vi "VI-File-Explorer_1.vi"() -> ()   [LabVIEW 2021, in "vi_lib.lvlib"]
uses:
  vi_lib.lvlib
  clLabview/clLabview.lvclass
  clFile/clFile.lvclass
panel:
  out "concatenated string":string
  in  "new VI-Lib Password":string
  in  "Update LV-Lib Password":bool
  out "File is protected?":bool=TRUE
  out "LV-Lib password (Hex)":string
  out "Icon":picture
  out "busy (*)":bool
  out "Salt (Hex)":string
  out "MD5-Hash 2 (Hex)":string
  out "MD5-Hash 1 (Hex)":string
  out "saving done":bool
  in  "save":bool
  in  "Open":bool
  in  "stop":bool
  out "flags":i32 step=1
  out "stage":u8(ring) items=["development", "alpha", "beta", "release"]
  out "build":u8 step=1
  out "bugfix":u8 step=1
  out "minor":u8 max=99 step=1
  out "major":u8=3 min=1 max=99 step=1
  out "version info":string
  out "version text":string
  in  "save to":path=path "D:/labview/file_in_(free).vi"
  in  "new File Password":string
  in  "open from":path=path "D:/labview/file.vi"
  out "MD5 password (Hex)":string
  # "MD5 password (Hex)\nMD5-Hash 1 (Hex)\nMD5-Hash 2 (Hex) for LV-Version >= 8\nLV-Lib password (Hex)"
  # "File password [BDPW]"
  # "for LV-Version >= 8"
  # "for LV-Version >= 12"
  # "File propertys [LVSR]"
  # "(*) This is a \"brute force\" version to calc the password Salt, \n      so it might take up to 30sec."
  # "File version [vers]"
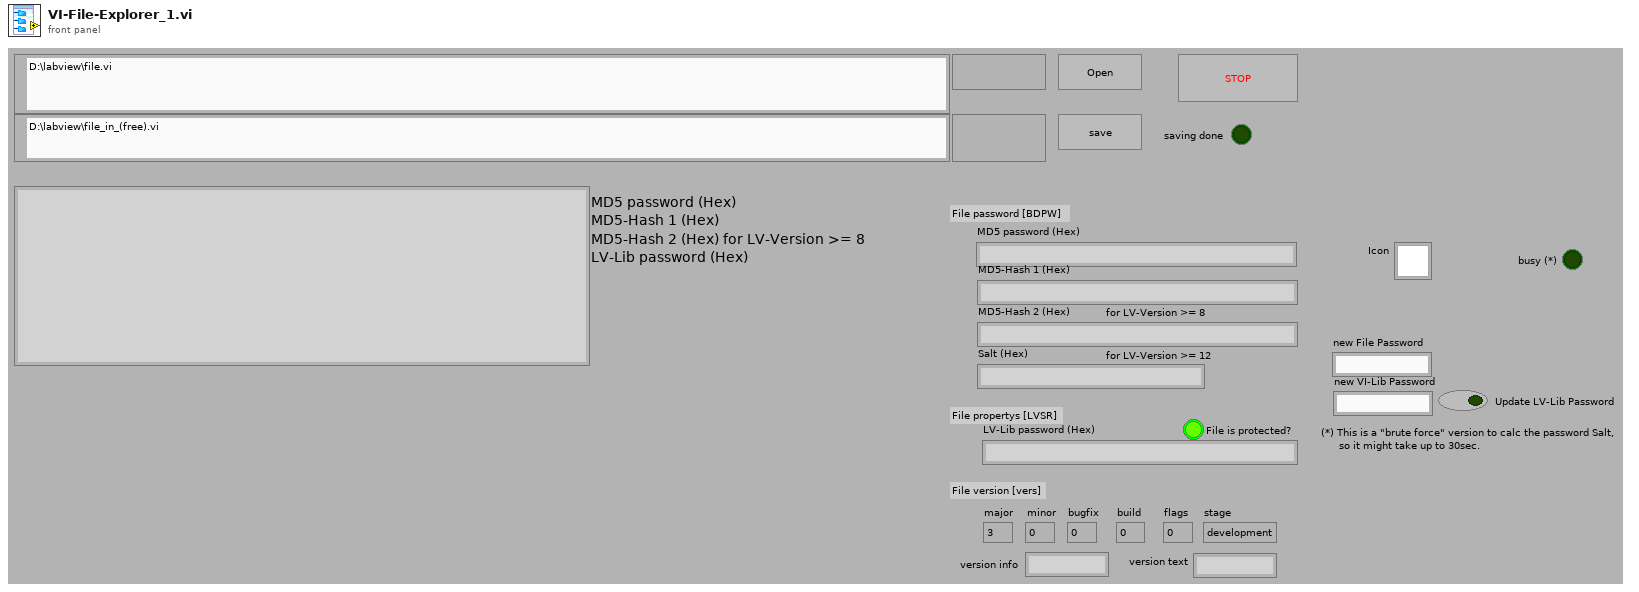
[diagram p1: front panel]
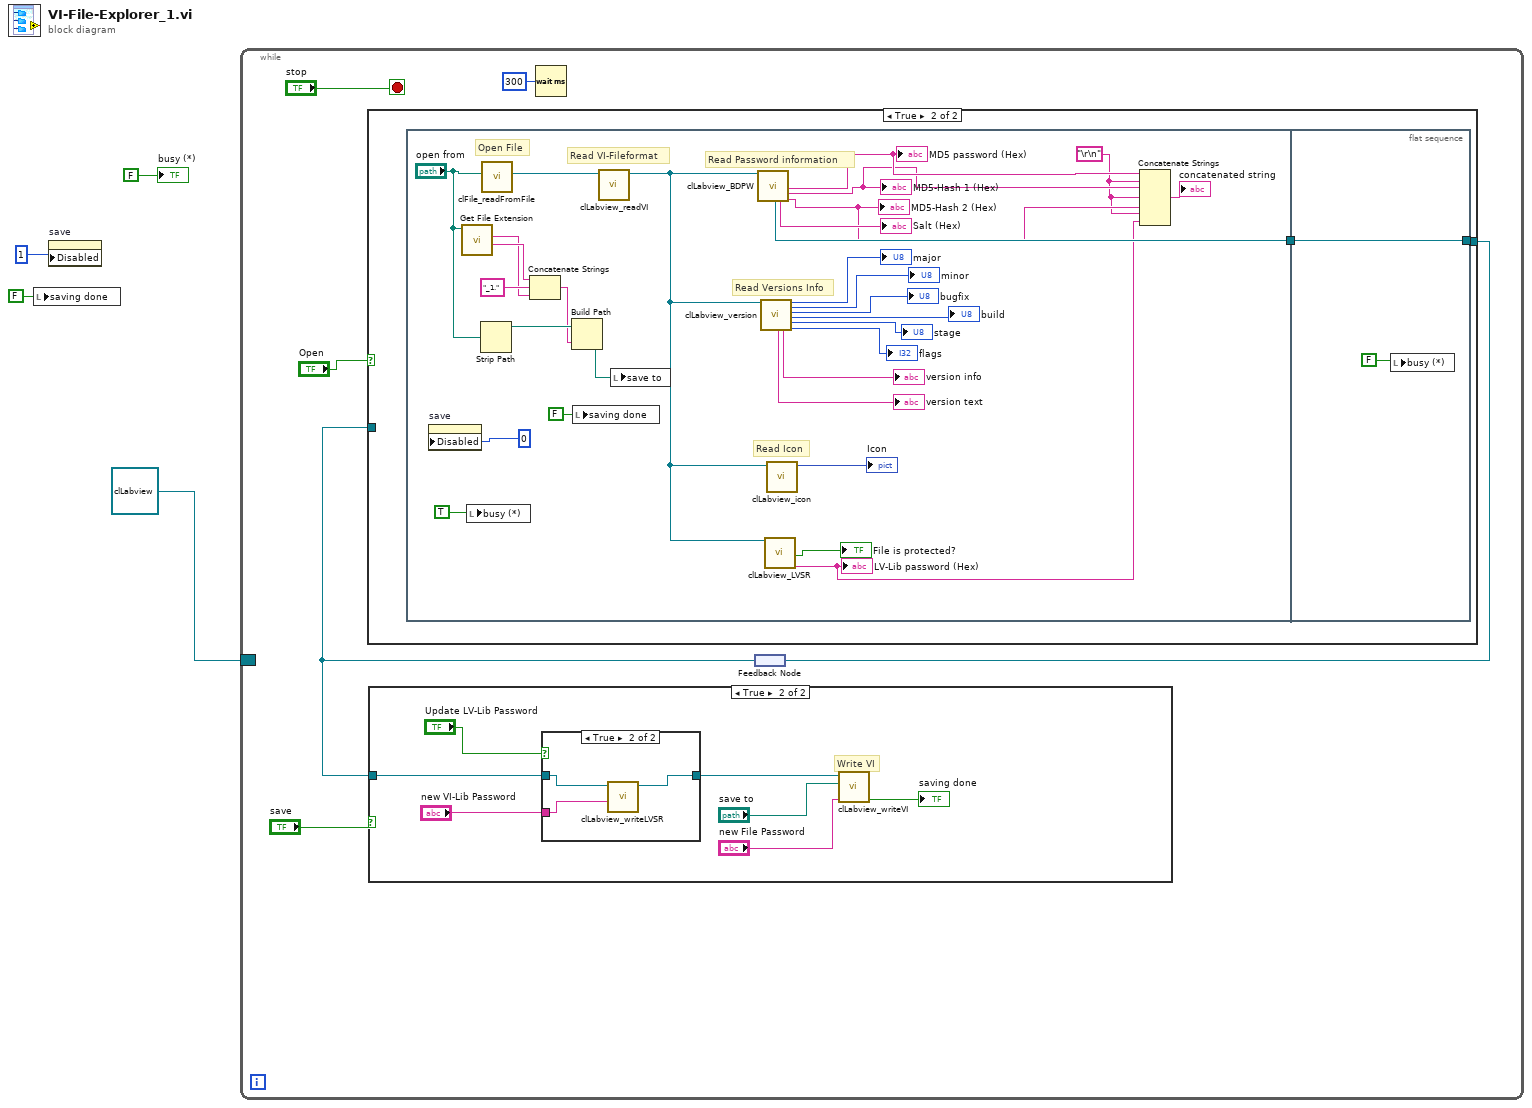
[diagram p0: block diagram]
diagram:
  n1 = local write "saving done"(FALSE ("saving done")) -> ()
  n2 = property on="save" class="Bool"("Disabled"=u8 1) -> ()  [unwired: 2 in, 2 out]
  n3 = while {
    border: refnum<class "clLabview.lvclass"> refnum ("vi_lib.lvlib:clLabview.lvclass 2") -> [_]
    stop <- "stop" stop-if-true
    n4 = Wait (ms)(milliseconds to wait=u32 300) -> ()  [unwired: 1 out]
    n5 = feedback #1() -> (w6:refnum<class "clLabview.lvclass">)
    n6 = case shown="True" "Open" {
      tunnel: [w22 w24] -> w8
      tunnel: w6 -> [w22 _]
      frame False {
      }
      frame True {
        n7 = flat-sequence {
          tunnel: [w43] -> w23
          tunnel: [w56] -> w24
          tunnel: w23 -> [w56]
          frame #0 {
            w27 = "\r\n"
            # "Read Icon"
            # "Read Versions Info"
            # "Read Password information"
            # "Read VI-Fileformat"
            # "Open File"
            n8 = property on="save" class="Bool"("Disabled"=u8 0) -> ()  [unwired: 2 in, 2 out]
            n9 = call <vilib>:"Get File Extension.vi"("file"="open from") -> ("filename without extension"=w35:string, "lowercase file extension"=w33:string)  [unwired: 6 in, 3 out]
            n10 = local write "busy (*)"(TRUE ("busy")) -> ()
            n11 = Strip Path(path="open from") -> (stripped path=w37:path)  [unwired: 1 out]
            n12 = call "clFile_readFromFile.vi"("file (use dialog)"="open from") -> ("clFileReader.lvclass"=w54:refnum<class "clFileReader.lvclass">)  [unwired: 1 in, 9 out]
            n13 = Concatenate Strings(w35, "_1." ("string"), w33) -> (w32:string)
            n14 = Build Path(base path=w37, name or relative path=w32) -> (appended path=w36:path)
            n15 = local write "saving done"(FALSE ("saving done")) -> ()
            n16 = call "clLabview_readVI.vi"("vi_lib.lvlib:clFileReader.lvclass"=w54) -> ("vi_lib.lvlib:clLabview.lvclass 2"=w40:refnum<class "clLabview.lvclass">)  [unwired: 10 out]
            n17 = local write "save to"(w36) -> ()
            n18 = call "clLabview_BDPW.vi"("vi_lib.lvlib:clLabview.lvclass"=w40) -> ("vi_lib.lvlib:clLabview.lvclass [Out]"=w43:refnum<class "clLabview.lvclass">, "Salt (Hex)"=→"Salt (Hex)":string, "MD5 password (Hex)"=w31:string, "MD5-Hash 1  (Hex)"=w30:string, "MD5-Hash 2  (Hex)"=w29:string)  [unwired: 14 out]
            "MD5 password (Hex)" <- w31
            "MD5-Hash 2 (Hex)" <- w29
            "MD5-Hash 1 (Hex)" <- w30
            n19 = call "clLabview_version.vi"("vi_lib.lvlib:clLabview.lvclass"=w40) -> ("version_text"=→"version text":string, "version_info"=→"version info":string, "major"=→"major":u8, "minor"=→"minor":u8, "bugfix"=→"bugfix":u8, "build"=→"build":u8, "stage"=→"stage":u8, "flags"=→"flags":i32)  [unwired: 11 out]
            n20 = call "clLabview_LVSR.vi"("vi_lib.lvlib:clLabview.lvclass"=w40) -> ("File is protected?"=→"File is protected?":bool, "MD5 lib Password (Hex)"=w26:string)  [unwired: 17 out]
            "LV-Lib password (Hex)" <- w26
            n21 = call "clLabview_icon.vi"("vi_lib.lvlib:clLabview.lvclass"=w40) -> ("Icon"=→"Icon":picture)  [unwired: 10 out]
            n22 = Concatenate Strings(w31, w27, w30, w27, w29, w27, w26) -> (→"concatenated string":string)
          }
          frame #1 {
            n23 = local write "busy (*)"(FALSE ("busy")) -> ()
          }
        }
      }
    }
    n24 = case shown="True" "save" {
      tunnel: w6 -> [_ w13]
      frame False {
      }
      frame True {
        # "Write VI"
        n25 = case shown="True" "Update LV-Lib Password" {
          tunnel: w13 -> [w18 w21]
          tunnel: [w18 w20] -> w14
          tunnel: "new VI-Lib Password" -> [_ w19]
          frame False {
          }
          frame True {
            n26 = call "clLabview_writeLVSR.vi"("vi_lib.lvlib:clLabview.lvclass"=w21, "new lib Password"=w19) -> ("vi_lib.lvlib:clLabview.lvclass [Out]"=w20:refnum<class "clLabview.lvclass">)  [unwired: 8 out]
          }
        }
        n27 = call "clLabview_writeVI.vi"("vi_lib.lvlib:clLabview.lvclass"=w14, "filename (use dialog)"="save to", "new Password"="new File Password") -> ("no Error"=→"saving done":bool)  [unwired: 7 out]
      }
    }
    n28 = feedback-in #1(w8) -> ()
  }
  "busy (*)" <- FALSE ("busy")
